vi "Read Relay Name.vi"(8 "error in (no error)":errorcluster, 11 "SwitchMatrix in":refnum<class "SwitchMatrix.lvclass">) -> (0 "error out":errorcluster, 2 "Relay Name":string[](array[string]), 3 "SwitchMatrix out":refnum<class "SwitchMatrix.lvclass">)   [LabVIEW 2019, in "SwitchMatrix.lvlib" / "SwitchMatrix.lvclass"]
uses:
  Library/SwitchMatrix.lvclass
  Library/SwitchMatrix.lvclass/SwitchMatrix.ctl
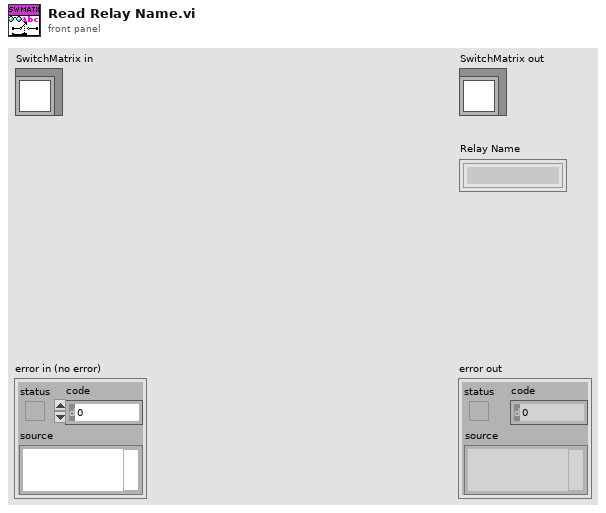
[diagram p1: front panel]
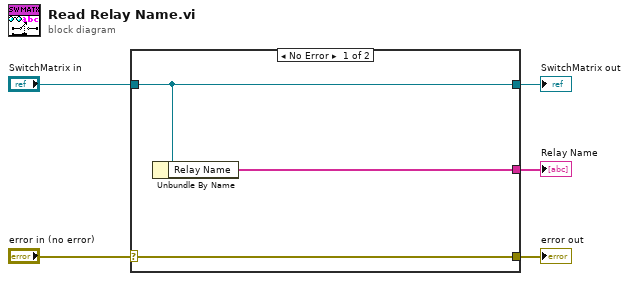
[diagram p0: block diagram]
diagram:
  n1 = case shown="No Error" "error in (no error)" {
    selector: "error in (no error)" -> [w8 w9]
    tunnel: [w8 w9] -> w4
    tunnel: [w7 w10] -> w2
    tunnel: "SwitchMatrix in" -> [w7 w10]
    tunnel: [w6 _] -> w1
    frame No Error {
      n2 = Unbundle By Name(w7) -> ("Relay Name"=w6:string[])
    }
    frame Error {
    }
  }
  "error out" <- w4
  "SwitchMatrix out" <- w2
  "Relay Name" <- w1
